vi "SetGenericFeedback.vi"(0 "Generic Feedback Cluster":T1={"Number"=0, "P"=-2147483600.0, "Input Channel"=-2147483648, "I"=-2147483648, "Output Channel"=-2147483648, "Setpoint [a.u.]"=-inf, "Min"=-2147483600.0, "Invert Polarity"=-2147483648, "Max"=-2147483600.0, "Transfer function"=FALSE} {"Max" format="%#_g V"; "Invert Polarity" items=["[read only]"=-2147483648, "No"=0, "Yes"=1]; "Min" format="%#_g V"; "Output Channel" items=["[read only]"=-2147483648, "DAC 1"=0, "DAC 2"=1, "DAC 3"=2, "DAC 4"=3]; "I" format="%.0f mHz"; "Input Channel" items=["[read only]"=-2147483648, "ADC 1"=0, "ADC 2"=1, "ADC 3"=2, "ADC 4"=3, "ADC 5"=4, "ADC 6"=5, "HF 1 df "=8, "HF 1 Ampl"=13, "HF 1 Phase"=14, "LF LockIn Ampl"=16, "LF LockIn Phase"=17, "Counter"=23]; "Number" items=["1", "2"]}, 5 "error in":T6) -> (14 "Output Cluster":T1={"Number"=0, "P"=-2147483600.0, "Input Channel"=-2147483648, "I"=-2147483648, "Output Channel"=-2147483648, "Setpoint [a.u.]"=-inf, "Min"=-2147483600.0, "Invert Polarity"=-2147483648, "Max"=-2147483600.0, "Transfer function"=FALSE} {"Max" format="%#_g V"; "Invert Polarity" items=["[read only]"=-2147483648, "No"=0, "Yes"=1]; "Min" format="%#_g V"; "Output Channel" items=["[read only]"=-2147483648, "DAC 1"=0, "DAC 2"=1, "DAC 3"=2, "DAC 4"=3]; "I" format="%.0f mHz"; "Input Channel" items=["[read only]"=-2147483648, "ADC 1"=0, "ADC 2"=1, "ADC 3"=2, "ADC 4"=3, "ADC 5"=4, "ADC 6"=5, "HF 1 df "=8, "HF 1 Ampl"=13, "HF 1 Phase"=14, "LF LockIn Ampl"=16, "LF LockIn Phase"=17, "Counter"=23]; "Number" items=["1", "2"]}, 19 "error out":T6)   [LabVIEW 2016]
doc: "This VI changes the settings for a generic feedback. The cluster includes:\n\n- Number (integer) [0 -- crosslink 1; 1 -- crosslink 2] (required input)\n- Input Channel (integer) [0-5 -- ADC1-6; 8 -- AFM df; 13 -- AFM Aosc; 14 -- AFM Phase; 16 -- LockIn Ampl; 17 -- LockIn Phase]\n- Output Channel (integer) [0-3 -- DAC1-4]\n- Min in V (float) [without restraint]\n- Max in V (float) [without restraint]\n- P (float) [0 to 100]\n- I in mHz (integer) [without restraint]\n- Setpoint: Unit depends on \"Input Channel\": mV, Hz or degree (float) [without restraint]\n- Invert Polarity (integer) [0 -- no; 1 -- yes]\nBy passing -Inf (float) or -2147483648 (integer) as input values, the corresponding parameter(s) will be read out."
uses:
  Controls/Generic-Feedback_Parameters.ctl
  Controls/Generic-Feedback-Number_Selection.ctl
  Controls/Generic-Feedback-Input-Channel_Selection.ctl
  Controls/Generic-Feedback-Output-Channel_Selection.ctl
  Controls/Invert-Polarity_Selection.ctl
  Controls/Error_Out.ctl
  Files_ASC500/DLL/ASC500_RemoteControlV27.dll
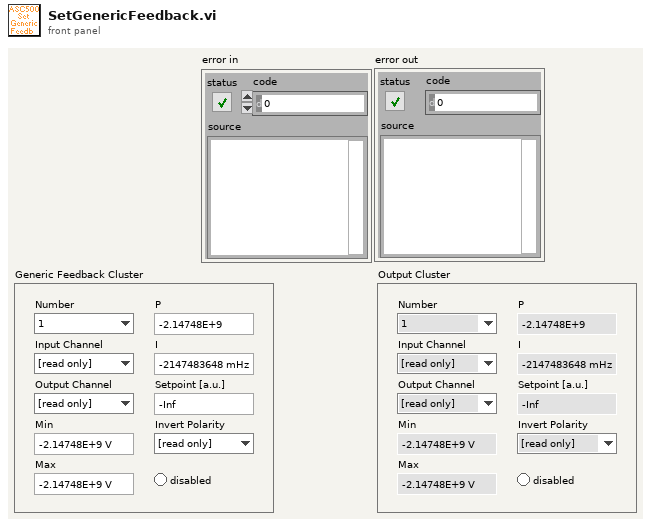
[diagram p1: front panel]
types:
  T1 = typedef "Generic-Feedback_Parameters.ctl" = cluster{"Number":T2, "P":sgl, "Input Channel":T3, "I":i32, "Output Channel":T4, "Setpoint [a.u.]":sgl, "Min":sgl, "Invert Polarity":T5, "Max":sgl, "Transfer function":bool}
  T2 = typedef "Generic-Feedback-Number_Selection.ctl" = i32
  T3 = typedef "Generic-Feedback-Input-Channel_Selection.ctl" = i32
  T4 = typedef "Generic-Feedback-Output-Channel_Selection.ctl" = i32
  T5 = typedef "Invert-Polarity_Selection.ctl" = i32
  T6 = typedef "Error_Out.ctl" = errorcluster
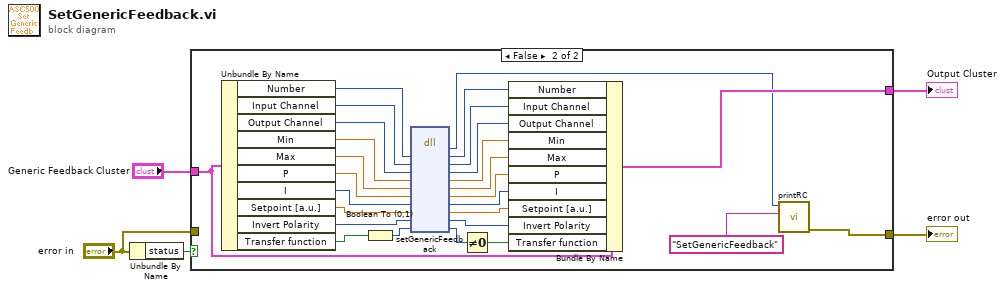
[diagram p0: block diagram]
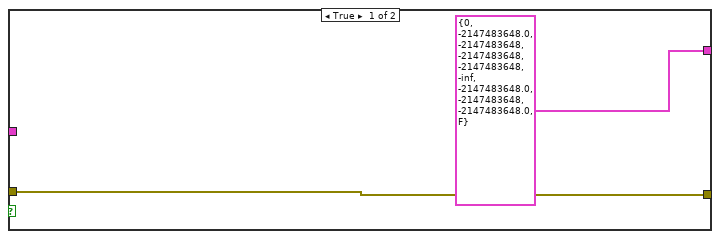
[diagram p2: hidden frame]
diagram:
  n1 = Unbundle By Name("error in") -> ("status"=w5:bool)
  n2 = case shown="False" w5 {
    tunnel: [w6 w14] -> w4
    tunnel: "Generic Feedback Cluster" -> [_ w16]
    tunnel: [T1 {"Number"=0, "P"=-2147483600.0, "Input Channel"=-2147483648, "I"=-2147483648, "Output Channel"=-2147483648, "Setpoint [a.u.]"=-inf, "Min"=-2147483600.0, "Invert Polarity"=-2147483648, "Max"=-2147483600.0, "Transfer function"=FALSE} ("Generic Feedback Cluster") w15] -> w2
    tunnel: "error in" -> [w6 _]
    frame True {
    }
    frame False {
      n3 = Unbundle By Name(w16) -> ("Number"=w34:T2, "Input Channel"=w33:T3, "Output Channel"=w32:T4, "Min"=w31:sgl, "Max"=w30:sgl, "P"=w29:sgl, "I"=w28:i32, "Setpoint [a.u.]"=w27:sgl, "Invert Polarity"=w26:T5, "Transfer function"=w10:bool)
      n4 = Boolean To (0,1)(Boolean=w10) -> (0, 1=w11:i16)
      n5 = dll-call lib="G:/SCMOperations/Share/ELE/Produkt Information/ASC500/04 Remote Control/02 development versions/2018Nov06/Files_ASC500/DLL/ASC500_RemoteControlV27.dll" fn="setGenericFeedback"("Number"=w34, "Input Channel"=w33, "Output Channel"=w32, "Min"=w31, "Max"=w30, "P"=w29, "I"=w28, "Setpoint"=w27, "Invert Polarity"=w26, "state"=w11) -> ("return type"=w13:i32, "Number"=w17:i32, "Input Channel"=w18:i32, "Output Channel"=w19:i32, "Min"=w25:sgl, "Max"=w24:sgl, "P"=w23:sgl, "I"=w22:i32, "Setpoint"=w21:sgl, "Invert Polarity"=w20:i32, "state"=w9:i32)  [unwired: 3 in, 2 out]
      n6 = Not Equal To 0?(x=w9) -> (x != 0?=w8:bool)
      n7 = Bundle By Name(cluster=w16, "Number"=w17, "Input Channel"=w18, "Output Channel"=w19, "Min"=w25, "Max"=w24, "P"=w23, "I"=w22, "Setpoint [a.u.]"=w21, "Invert Polarity"=w20, "Transfer function"=w8) -> (w15:T1)
      n8 = call "printRC.vi"("additional information"="SetGenericFeedback", "RC"=w13) -> ("error out"=w14:T6)  [unwired: 9 in]
    }
  }
  "error out" <- w4
  "Output Cluster" <- w2
